vi "Send Log Data.vi"(8 "error in":errorcluster, 10 "Data":T1[](array[typedef]), 11 "Log Producer in":refnum<class "Log Producer.lvclass">) -> (0 "error out":errorcluster, 3 "Log Producer out":refnum<class "Log Producer.lvclass">)   [LabVIEW 2020, in "AIM ARINC 429 Engine.lvlib" / "Implementation.lvlib" / "Word Logging.lvlib" / "Log Producer.lvclass"]
uses:
  Log Producer.lvclass
  Word.ctl
  Log Producer.lvclass/Log Producer.ctl
  Log Message/Log Message.lvclass
  C:/Program Files (x86)/National Instruments/LabVIEW 2020/vi.lib/NI/VeriStand Custom Device Messaging/Message/Abstract Message/Abstract Message.lvclass
  Implementation.lvlib
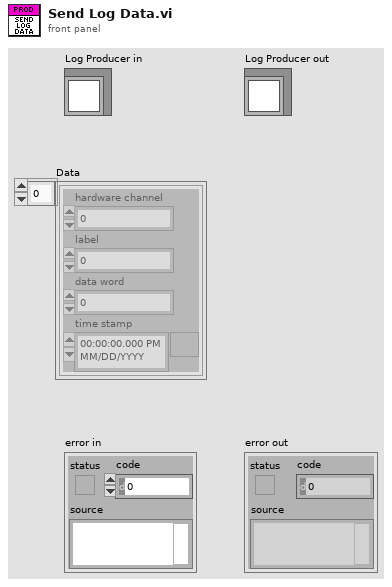
[diagram p1: front panel]
types:
  T1 = typedef "AIM ARINC 429 Engine.lvlib/Implementation.lvlib/Word.ctl" = cluster{"hardware channel":u8, "label":u8, "data word":u32, "time stamp":timestamp}
  T2 = typedef "AIM ARINC 429 Engine.lvlib/Implementation.lvlib/Word Logging.lvlib/Logger Data Reference.ctl" = refnum<data-value>
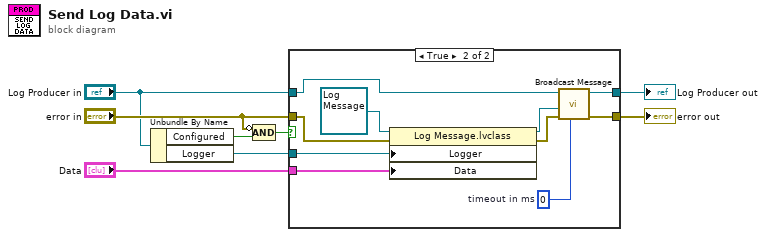
[diagram p0: block diagram]
diagram:
  n1 = Unbundle By Name("Log Producer in") -> ("Configured"=w2:bool, "Logger"=w3:T2)
  n2 = Compound Arithmetic op=AND(invert "error in", w2) -> (w1:bool)
  n3 = case shown="True" w1 {
    tunnel: w3 -> [_ w20]
    tunnel: "error in" -> [w9 w13]
    tunnel: [w9 w19] -> w7
    tunnel: "Log Producer in" -> [w10 w11]
    tunnel: [w10 w18] -> w5
    tunnel: "Data" -> [_ w15]
    frame False {
    }
    frame True {
      w14 = 0  # timeout in ms
      n4 = property class="Log Message.lvclass"(reference=refnum<class "Log Message.lvclass"> refnum ("Communication Bus Template Interfaces:Implementation.lvlib:Logging.lvlib:Log Word Message.lvclass"), error in=w13, "Logger"=w20, "Data"=w15) -> (reference out=w17:refnum<class "Log Message.lvclass">, error out=w12:errorcluster)
      n5 = call-dynamic "Broadcast Message.vi"("timeout in ms (-1)"=w14, "error in (no error)"=w12, "Message in"=w17, "Abstract Producer in"=w11) -> ("error out"=w19:errorcluster, "Abstract Producer out"=w18:refnum<class "Log Producer.lvclass">)  [unwired: 4 in, 2 out]
    }
  }
  "error out" <- w7
  "Log Producer out" <- w5
